vi "ASI Set Start Pos.vi"(9 "iStartY":i32, 10 "iStartX":i32, 11 "iCameraID":i32) -> (3 "function return":i32)   [LabVIEW 2012, in "ASICamera2_no_err.lvlib"]
doc: "ASICAMERA_API ASI_ERROR_CODE ASISetStartPos(int iCameraID, int iStartX, int iStartY);"
uses:
  <userlib>/ASICamera2_no_err/ASICamera2_no_err.lvlib
  ASICamera2.dll
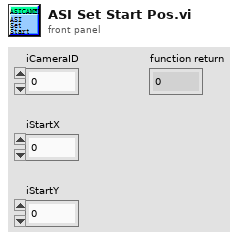
[diagram p1: front panel]
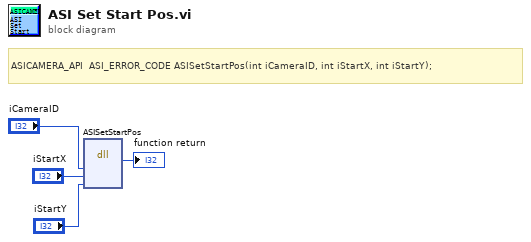
[diagram p0: block diagram]
diagram:
  # "ASICAMERA_API  ASI_ERROR_CODE ASISetStartPos(int iCameraID, int iStartX, int iStartY);"
  n1 = dll-call lib="ASICamera2.*" fn="ASISetStartPos"("iCameraID"="iCameraID", "iStartX"="iStartX", "iStartY"="iStartY") -> (→"function return":i32)  [unwired: 6 in, 2 out]
